vi "Open FPGA Ref.vi"(8 "error in (no error)":errorcluster, 10 "Bitfile Path":path, 11 "Device address":string) -> (0 "error out":errorcluster, 3 "FPGA Ref out":refnum<k20>)   [LabVIEW 2025]
uses:
  <vilib>/FPGAPlugInAG/Dynamic/niLvFpga_Close_Dynamic.vi
  <vilib>/rvi/interface/nirviCloseFPGA/nirviCloseFPGA.xnode
  <instrlib>/FlexRIO/API/Host/v1/NI FlexRIO API v1.lvlib
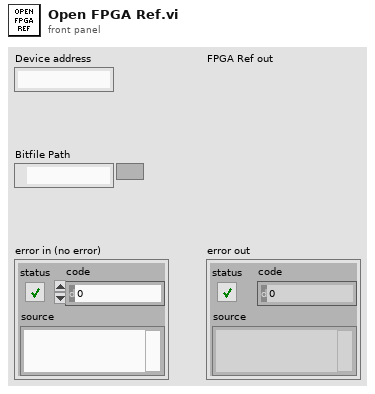
[diagram p1: front panel]
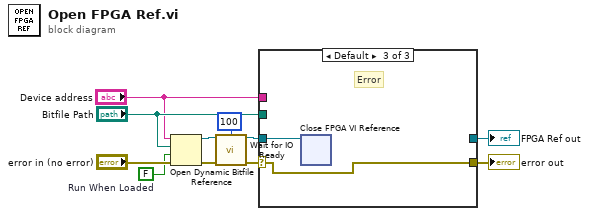
[diagram p0: block diagram]
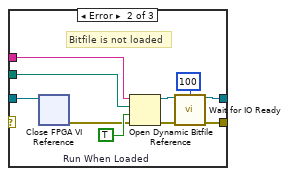
[diagram p3: hidden frame]
diagram:
  w4 = FALSE  # Run When Loaded
  n1 = Open Dynamic Bitfile Reference(0:"Device address", 1:"Bitfile Path", 2:w4, 3:"error in (no error)") -> (5:w2:refnum<k20>, 8:w3:errorcluster)  [unwired: 1 in]
  n2 = call <instrlib>:"Wait for IO Ready.vi"("fpga interface in"=w2, "timeout"=100, "error in"=w3) -> ("fpga interface out"=w7:refnum<k20>, "error out"=w6:errorcluster)  [unwired: 9 in, 2 out]
  n3 = case shown="Default" w6 {
    selector: w6 -> [w13 _ w24]
    tunnel: [w13 w15 w24] -> w10
    tunnel: w7 -> [w12 w23 w25]
    tunnel: "Device address" -> [_ w17 _]
    tunnel: "Bitfile Path" -> [_ w16 _]
    tunnel: [w12 w14 _] -> w11
    frame No Error {
      # "Bitfile is loaded"
    }
    frame Error {
      w19 = TRUE  # Run When Loaded
      # "Bitfile is not loaded"
      n4 = xnode ("Close FPGA VI Reference")("FPGA VI Reference In"=w23) -> ("error out"=w18:errorcluster)  [unwired: 1 in]
      n5 = Open Dynamic Bitfile Reference(0:w17, 1:w16, 2:w19, 3:w18) -> (5:w21:refnum<k20>, 8:w20:errorcluster)  [unwired: 1 in]
      n6 = call <instrlib>:"Wait for IO Ready.vi"("fpga interface in"=w21, "timeout"=100, "error in"=w20) -> ("fpga interface out"=w14:refnum<k20>, "error out"=w15:errorcluster)  [unwired: 9 in, 2 out]
    }
    frame Default {
      # "Error"
      n7 = xnode ("Close FPGA VI Reference")("FPGA VI Reference In"=w25) -> ()  [unwired: 1 in, 1 out]
    }
  }
  "FPGA Ref out" <- w11
  "error out" <- w10
